vi "FTW-ERR-ThrowError.vi"(7 "Error Message":string, 9 "Error Code":i32, 11 "error in":errorcluster, 13 "Source Level":i32 caption="Source Level (0 = This VI's caller)") -> (15 "error out":errorcluster)   [LabVIEW 2018]
doc: "Throws an error if the \"Error Code\" input is non-zero."
panel:
  # "Inputs"
  # "Outputs"
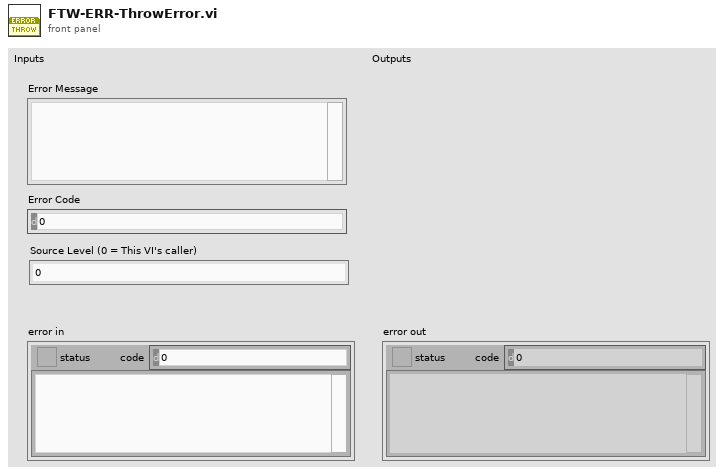
[diagram p1: front panel]
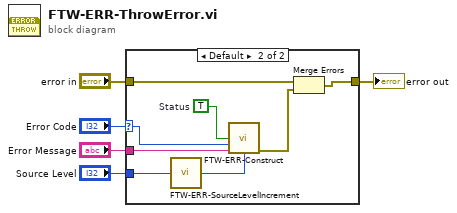
[diagram p0: block diagram]
diagram:
  n1 = case shown="Default" "Error Code" {
    selector: "Error Code" -> [_ w11]
    tunnel: "error in" -> [w6 w14]
    tunnel: [w6 w13] -> w4
    tunnel: "Error Message" -> [_ w10]
    tunnel: "Source Level" -> [_ w9]
    frame 0 {
    }
    frame Default {
      w12 = TRUE  # Status
      n2 = call "FTW-ERR-SourceLevelIncrement.vi"("SourceLevelIn"=w9) -> ("SourceLevelOut"=w7:i32)
      n3 = call "FTW-ERR-Construct.vi"("Status"=w12, "Error Code"=w11, "Error Message"=w10, "Source Level"=w7) -> ("error out"=w8:errorcluster)  [unwired: 11 in]
      n4 = Merge Errors(w14, w8) -> (w13:errorcluster)
    }
  }
  "error out" <- w4
